vi "rs3 run_onchip_calibration.vi"(6 "On-Chip Calibration Speed":T1(ring)=enum."Fast (Default)", 7 "Linux/Windows":u16(ring) items=["Linux (poling)", "Windows (interrupt)"], 8 "error in (no error)":errorcluster, 9 "On-Chip Calibration Mode":u16(ring) items=["Intrinsic", "Extrinsic"], 10 "timeout, ms":i32=4000, 11 "Device in":u64=2439423724432) -> (0 "error out":errorcluster, 1 "error":u64=2437885894512, 2 "health-check":sgl, 3 "Device out":u64=2439423724432, 4 "PointerToNewCalibrationTable":u64)   [LabVIEW 2017, in "libRealSense3.lvlib"]
doc: "STARTS the streaming of a specific sensor, based on the input QUEUE."
uses:
  libRealSense3.lvlib
  realsense2.dll
panel:
  out "json":string="{speed: 4, scan_parameter:0, data_sampling:0}"
  # "RS Run On-Chip Calibration"
  # "(C) 2019 Intel Corp.,  AGJ"
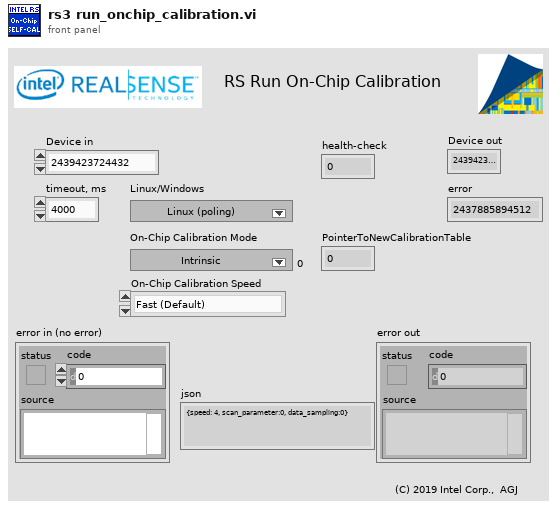
[diagram p1: front panel]
types:
  T1 = enum16{"Very Fast", "Fast (Default)", "Medium", "Slow", "White Wall"}
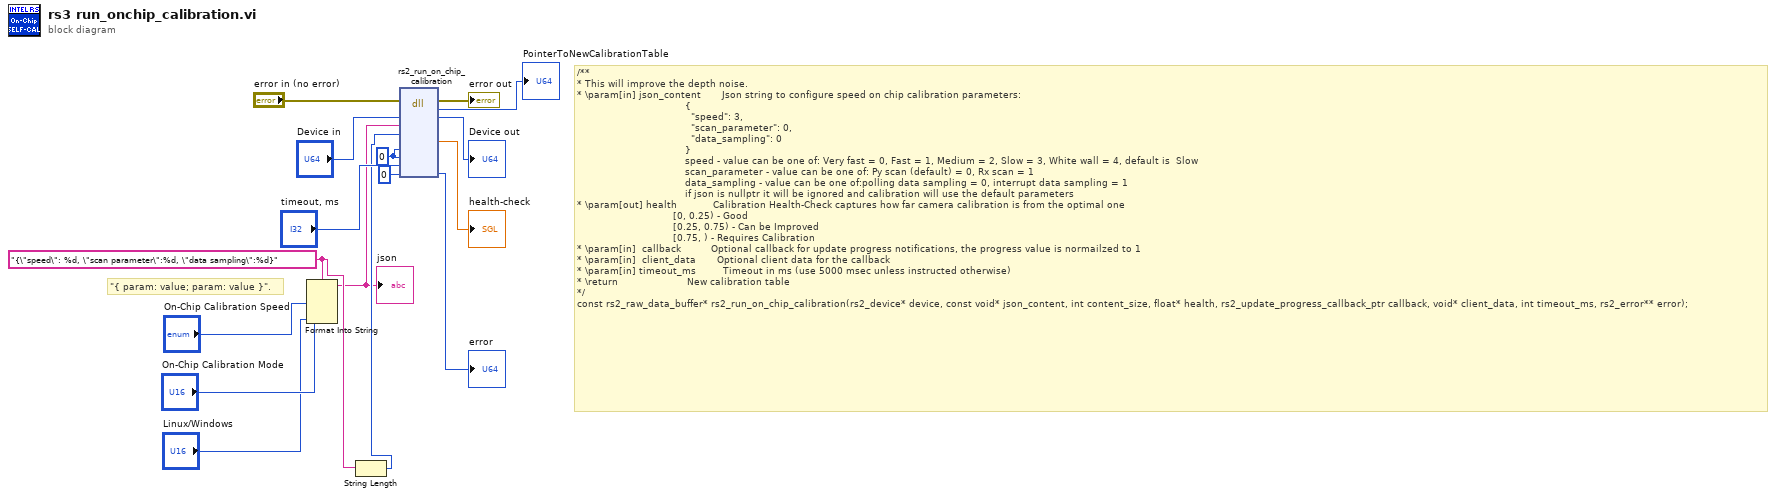
[diagram p0: block diagram]
diagram:
  w5 = "{\"speed\": %d, \"scan parameter\":%d, \"data sampling\":%d}" ("format string")
  w4 = u64 0 ("callback progress")
  # "/**\n* This will improve the depth noise.\n* \\param[in] json_content       Json string to configure speed on chip calibration parameters:\n                                    {\n                                      \"speed\": 3,\n                                      \"scan_parameter\": 0,\n                                      \"data_sampling\": 0\n                                    }\n                                    speed - value can be one of: Very fast = 0, Fast = 1, Medium = 2, Slow = 3, White wall = 4, default is  Slow\n                                    scan_parameter - value can be one of: Py scan (default) = 0, Rx scan = 1\n                                    data_sampling - value can be one of:polling data sampling = 0, interrupt data sampling = 1\n                                    if json is nullptr it will be ignored and calibration will use the default parameters\n* \\param[out] health            Calibration Health-Check captures how far camera calibration is from the optimal one\n                                [0, 0.25) - Good\n                                [0.25, 0.75) - Can be Improved\n                                [0.75, ) - Requires Calibration\n* \\param[in]  callback          Optional callback for update progress notifications, the progress value is normailzed to 1\n* \\param[in]  client_data       Optional client data for the callback\n* \\param[in] timeout_ms         Timeout in ms (use 5000 msec unless instructed otherwise)\n* \\return                       New calibration table\n*/\nconst rs2_raw_data_buffer* rs2_run_on_chip_calibration(rs2_device* device, const void* json_content, int content_size, float* health, rs2_update_progress_callback_ptr callback, void* client_data, int timeout_ms, rs2_error** error);"
  # "\"{ param: value; param: value }\"."
  n1 = Format Into String(format string=w5, "On-Chip Calibration Speed", "On-Chip Calibration Mode", "Linux/Windows") -> (resulting string=w2:string)  [unwired: 2 in, 1 out]
  "json" <- w2
  n2 = String Length(string=w5) -> (length=w3:i32)
  n3 = dll-call lib="C:/Users/agrunnet/Documents/libRealSense6/realsense2.dll" fn="rs2_run_on_chip_calibration"(error in="error in (no error)", "device"="Device in", "json"=w2, "json content size"=w3, "callback progress"=w4, "client_data"=w4, "timeout"="timeout, ms", "error"=u64 0) -> (error out=→"error out":errorcluster, "calibrationTable"=→"PointerToNewCalibrationTable":u64, "device"=→"Device out":u64, "health-check"=→"health-check":sgl, "error"=→"error":u64)  [unwired: 8 in, 1 out]
